vi "WebcamTest.vi"() -> ()   [LabVIEW 2013]
panel:
  out "Camera Image":T1(plugin-control)
  out "MatchFound?":bool
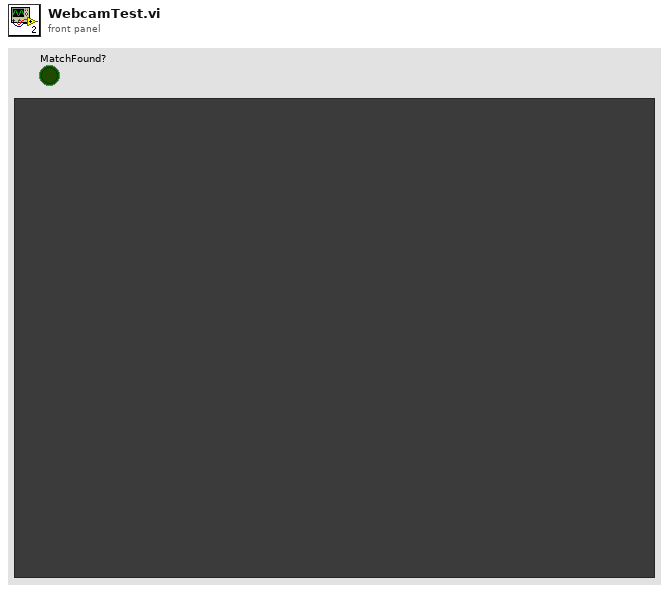
[diagram p1: front panel]
types:
  T1 = typedef "IMAQ Image.ctl" = refnum<image>
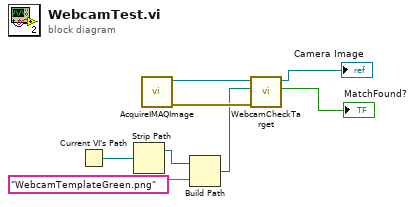
[diagram p0: block diagram]
diagram:
  n1 = Current VI's Path() -> (path=w3:path)
  n2 = Strip Path(path=w3) -> (stripped path=w2:path)  [unwired: 1 out]
  n3 = call "AcquireIMAQImage.vi"() -> ("error out"=w7:errorcluster, "ImageOut"=w8:T1)  [unwired: 10 in]
  n4 = Build Path(base path=w2, name or relative path="WebcamTemplateGreen.png") -> (appended path=w4:path)
  n5 = call "WebcamCheckTarget.vi"("error in"=w7, "TemplatePath"=w4, "ImageIn"=w8) -> ("MatchFound?"=→"MatchFound?":bool, "Image Out"=→"Camera Image":T1)  [unwired: 6 in, 1 out]
